vi "Create Session Ref(IL).vi"(8 "error in (no error)":errorcluster, 10 "interface":refnum<k21>, 11 "LDF Path":path) -> (0 "error out":errorcluster, 3 "LIN Device":T1={"Master Frame(3C)"="MasterReq\nSPA3414_ConfigurationsCMAGeely_CEMCALYPSOSDB34XX0Cfg_LIN3_190709_", "Slave Frame(3D)"="SlaveResp\nSPA3414_ConfigurationsCMAGeely_CEMCALYPSOSDB34XX0Cfg_LIN3_190709_", "Request Schedule"="CEMLIN3DiagRequestSchedule\nSPA3414_ConfigurationsCMAGeely_CEMCALYPSOSDB34XX0Cfg_LIN3_190709_", "Response Schedule"="CEMLIN3DiagResponseSchedule\nSPA3414_ConfigurationsCMAGeely_CEMCALYPSOSDB34XX0Cfg_LIN3_190709_", "Frame Write SCU"="", "Frame Read SCU"="", "LIN Name"=""})   [LabVIEW 2018]
uses:
  LIN Device.ctl
  <vilib>/xnet/xnet.llb/XNET Create Session (Frame Input Queued).vi
  <vilib>/xnet/xnet.llb/XNET Create Session (Frame Output Queued).vi
  <resource>/objmgr/xnet.rc
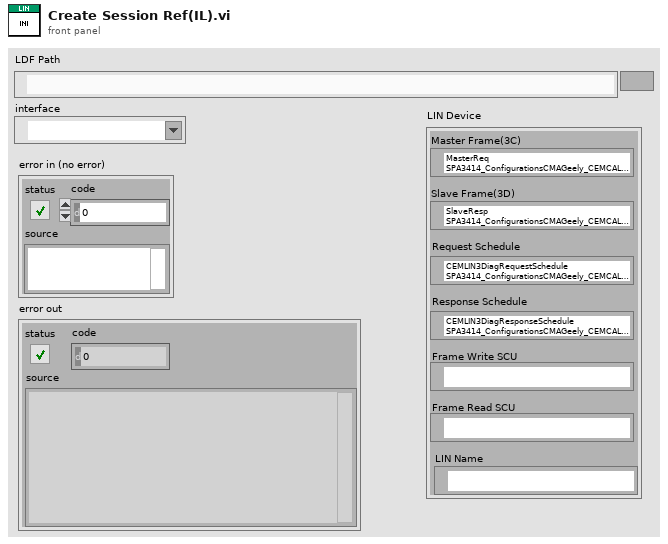
[diagram p1: front panel]
types:
  T1 = typedef "LIN Device.ctl" = cluster{"Master Frame(3C)":refnum<k21>, "Slave Frame(3D)":refnum<k21>, "Request Schedule":refnum<k21>, "Response Schedule":refnum<k21>, "Frame Write SCU":refnum<k21>, "Frame Read SCU":refnum<k21>, "LIN Name":refnum<k21>}
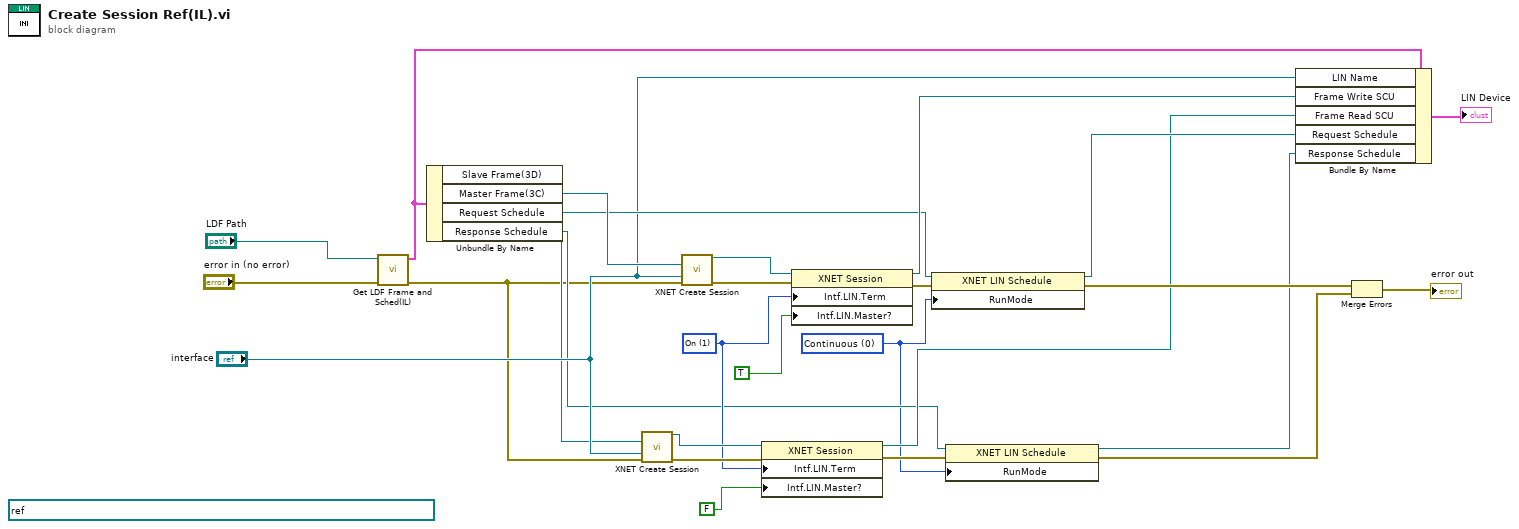
[diagram p0: block diagram]
diagram:
  (unwired) refnum<k21> "SPA3414_ConfigurationsCMAGeely_CEMCALYPSOSDB34XX0Cfg_LIN3" ("cluster (:memory:)")
  w6 = u32 0 items=["Continuous", "Once", "Null"] ("Run Mode")
  w12 = u32 1 items=["Off", "On"] ("Interface:LIN:Termination")
  n1 = call "Get LDF Frame and Sched(IL).vi"("error in (no error)"="error in (no error)", "LDF Path"="LDF Path") -> ("error out"=w2:errorcluster, "LIN Device"=w24:T1)  [unwired: 8 in]
  n2 = Unbundle By Name(w24) -> ("Slave Frame(3D)"=w3:refnum<k21>, "Master Frame(3C)"=w25:refnum<k21>, "Request Schedule"=w19:refnum<k21>, "Response Schedule"=w7:refnum<k21>)
  n3 = call-poly <vilib>:"XNET Create Session.vi"("frame"=w3, "interface"="interface", "error in (no error)"=w2) -> ("session out"=w13:refnum<k21>, "error out"=w14:errorcluster)  [unwired: 11 in]
  n4 = call-poly <vilib>:"XNET Create Session.vi"("frame"=w25, "interface"="interface", "error in (no error)"=w2) -> ("session out"=w22:refnum<k21>, "error out"=w23:errorcluster)  [unwired: 11 in]
  n5 = property class="XNET Session"(reference=w13, error in=w14, "Intf.LIN.Term"=w12, "Intf.LIN.Master?"=FALSE) -> (reference out=w10:refnum<k21>, error out=w8:errorcluster)
  n6 = property class="XNET Session"(reference=w22, error in=w23, "Intf.LIN.Term"=w12, "Intf.LIN.Master?"=TRUE ("Interface:LIN:Master?")) -> (reference out=w21:refnum<k21>, error out=w20:errorcluster)
  n7 = property class="XNET LIN Schedule"(reference=w19, error in=w20, "RunMode"=w6) -> (reference out=w18:refnum<k21>, error out=w16:errorcluster)
  n8 = property class="XNET LIN Schedule"(reference=w7, error in=w8, "RunMode"=w6) -> (reference out=w4:refnum<k21>, error out=w5:errorcluster)
  n9 = Bundle By Name(cluster=w24, "LIN Name"="interface", "Frame Write SCU"=w21, "Frame Read SCU"=w10, "Request Schedule"=w18, "Response Schedule"=w4) -> (→"LIN Device":T1)
  n10 = Merge Errors(w16, w5) -> (→"error out":errorcluster)
